vi "GUI.vi"() -> ()   [LabVIEW 2021, in "App-Builder Library.lvlib" / "Builder.lvclass"]
uses:
  Builder.lvclass
  Build Type.ctl
  App descriptions.ctl
panel:
  out "Next Version":string
  out "Current Version":string
  in  "Build all":bool
  out "Applications":T1[](array[typedef])
  in  "Build Type":T2
  # "-->"
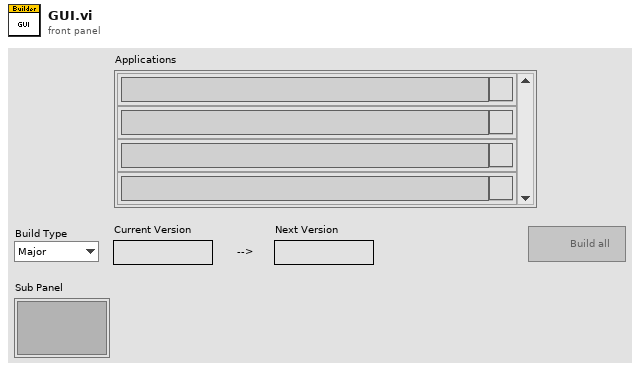
[diagram p1: front panel]
types:
  T1 = typedef "App-Builder Library.lvlib/Builder.lvclass/App descriptions.ctl" = cluster{"App Name":string, "Check":bool}
  T2 = typedef "App-Builder Library.lvlib/Builder.lvclass/Build Type.ctl" = enum16{"Major", "Minor", "Fix", "Build"}
  T3 = enum8{"Enabled", "Disabled", "Disabled and Grayed Out"}
  T4 = typedef "NI_App_Builder_API.lvlib/Build Specification Version.ctl" = cluster{"Major":u16, "Minor":u16, "Fix":u16, "Build":u16}
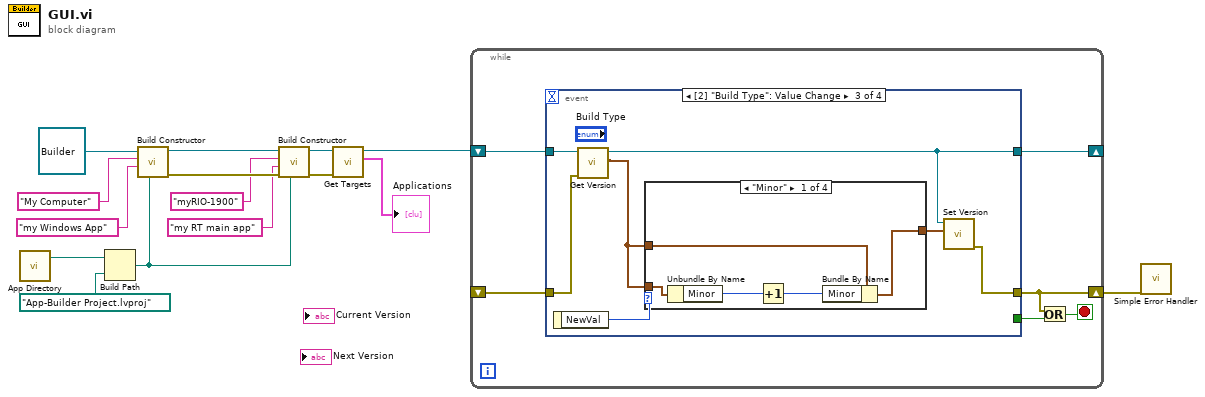
[diagram p0: block diagram]
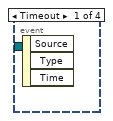
[diagram p2: hidden frame]
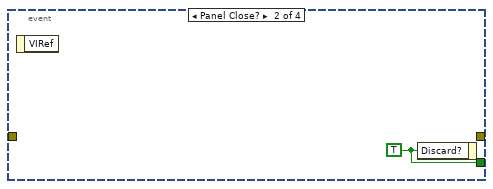
[diagram p3: hidden frame]
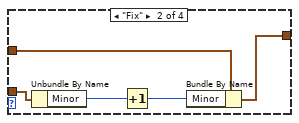
[diagram p4: hidden frame]
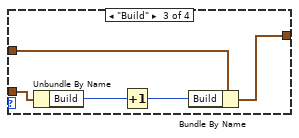
[diagram p5: hidden frame]
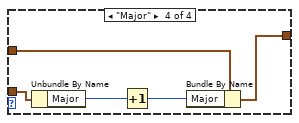
[diagram p6: hidden frame]
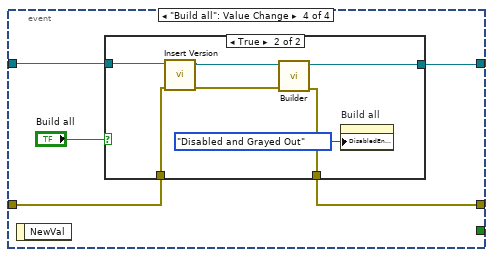
[diagram p7: hidden frame]
diagram:
  n1 = call "App Directory.vi"() -> ("App Directory"=w11:path)  [unwired: 11 in]
  n2 = Build Path(base path=w11, name or relative path=path "App-Builder Project.lvproj") -> (appended path=w1:path)
  n3 = call "Build Constructor.vi"("Project Path"=w1, "Build Specification"="my Windows App", "Target Name"="My Computer", "Builder in"=refnum<class "Builder.lvclass"> refnum ("App-Builder Library:Builder")) -> ("error out"=w12:errorcluster, "Builder out"=w5:refnum<class "Builder.lvclass">)  [unwired: 6 in]
  n4 = call "Build Constructor.vi"("Project Path"=w1, "error in (no error)"=w12, "Build Specification"="my RT main app", "Target Name"="myRIO-1900", "Builder in"=w5) -> ("error out"=w6:errorcluster, "Builder out"=w4:refnum<class "Builder.lvclass">)  [unwired: 5 in]
  n5 = call "Get Targets.vi"("error in (no error)"=w6, "Builder in"=w4) -> ("Applications"=→"Applications":T1[], "Builder out"=w13:refnum<class "Builder.lvclass">)  [unwired: 7 in, 1 out]
  n6 = while {
    shift-right: [w20] -> _
    shift-left: w13 -> [w21]
    shift-right: [w16] -> w7
    shift-left: _ -> [w19]
    stop <- w18 stop-if-true
    n7 = event shown="[2] \"Build Type\": Value Change" {
      selector: _ -> [_ _ _ _]
      dyn-events: _ -> [_ _ _ _]
      timeout: _ -> [_ _ _ _]
      tunnel: [_ w22 _ _] -> w17
      tunnel: w21 -> [_ _ w29 w54]
      tunnel: [_ _ w27 w53] -> w20
      tunnel: [_ _ w24 w51] -> w16
      tunnel: w19 -> [_ _ w23 w52]
      event Timeout {
        n8 = event-data() -> ()  [unwired: 1 in, 3 out]
      }
      event Panel Close? {
        w22 = TRUE ("Discard?")
        n9 = event-data() -> ()  [unwired: 1 in, 1 out]
        n10 = event-data("Discard?"=w22) -> ()  [unwired: 1 in, 1 out]
      }
      event Value Change {
        n11 = event-data() -> ("NewVal"=w28:T2)  [unwired: 1 in]
        n12 = call-dynamic "Get Version.vi"("error in (no error)"=w23, "Builder in"=w29) -> ("Build Version"=w25:T4, "Builder out"=w27:refnum<class "Builder.lvclass">)  [unwired: 7 in, 1 out]
        n13 = case shown="\"Minor\"" w28 {
          tunnel: [w32 w37 w42 w47] -> w26
          tunnel: w25 -> [w34 w39 w44 w49]
          tunnel: w25 -> [w33 w38 w43 w48]
          frame "Minor" {
            n14 = Unbundle By Name(w34) -> ("Minor"=w31:u16)
            n15 = Increment(x=w31) -> (x+1=w30:u16)
            n16 = Bundle By Name(cluster=w33, "Minor"=w30) -> (w32:T4)
          }
          frame "Fix" {
            n17 = Unbundle By Name(w39) -> ("Minor"=w36:u16)
            n18 = Increment(x=w36) -> (x+1=w35:u16)
            n19 = Bundle By Name(cluster=w38, "Minor"=w35) -> (w37:T4)
          }
          frame "Build" {
            n20 = Unbundle By Name(w44) -> ("Build"=w41:u16)
            n21 = Increment(x=w41) -> (x+1=w40:u16)
            n22 = Bundle By Name(cluster=w43, "Build"=w40) -> (w42:T4)
          }
          frame "Major" {
            n23 = Unbundle By Name(w49) -> ("Major"=w46:u16)
            n24 = Increment(x=w46) -> (x+1=w45:u16)
            n25 = Bundle By Name(cluster=w48, "Major"=w45) -> (w47:T4)
          }
        }
        n26 = call "Set Version.vi"("Build Version"=w26, "Builder in"=w27) -> ("error out"=w24:errorcluster)  [unwired: 8 in, 1 out]
      }
      event "Build all": Value Change {
        n27 = event-data() -> ()  [unwired: 1 in, 1 out]
        n28 = case shown="True" "Build all" {
          tunnel: w54 -> [w55 w58]
          tunnel: [w55 w63] -> w53
          tunnel: w52 -> [w56 w57]
          tunnel: [w56 w62] -> w51
          frame False {
          }
          frame True {
            n29 = call "Insert Version.vi"("error in (no error)"=w57, "Builder in"=w58) -> ("error out"=w60:errorcluster, "Builder out"=w59:refnum<class "Builder.lvclass">)  [unwired: 8 in]
            n30 = call "Builder.vi"("error in"=w60, "Builder in"=w59) -> ("error out"=w62:errorcluster, "Builder out"=w63:refnum<class "Builder.lvclass">)  [unwired: 7 in, 1 out]
            n31 = property on="Build all" class="Bool"("DisabledEnum"=T3."Disabled and Grayed Out" ("Disabled")) -> ()  [unwired: 2 in, 2 out]
          }
        }
      }
    }
    n32 = Or(x=w16, y=w17) -> (x .or. y?=w18:bool)
  }
  n33 = call <vilib>:"Simple Error Handler.vi"("error in (no error)"=w7) -> ()  [unwired: 4 in, 5 out]
